vi "Write FTDI.vi"(8 "error in (no error)":errorcluster, 10 "Write STR":string="\u0014", 11 "FTDI Handle In":u32) -> (0 "error out":errorcluster, 2 "FT_Status":u32(ring) items=["FT_OK", "FT_INVALID_HANDLE", "FT_DEVICE_NOT_FOUND", "FT_DEVICE_NOT_OPENED", "FT_IO_ERROR", "FT_INSUFFICIENT_RESOURCES", "FT_INVALID_PARAMETER", "FT_INVALID_BAUD_RATE", "FT_DEVICE_NOT_OPENED_FOR_ERASE", "FT_DEVICE_NOT_OPENED_FOR_WRITE", "FT_FAILED_TO_WRITE_DEVICE", "FT_EEPROM_READ_FAILED", "FT_EEPROM_WRITE_FAILED", "FT_EEPROM_ERASE_FAILED", "FT_EEPROM_NOT_PRESENT", "FT_EEPROM_NOT_PROGRAMMED", "FT_INVALID_ARGS", "FT_NOT_SUPPORTED", "FT_OTHER_ERROR"], 3 "FTDI Handle Out":u32)   [LabVIEW 2011, in "NMR.lvclass"]
uses:
  NMR.lvclass
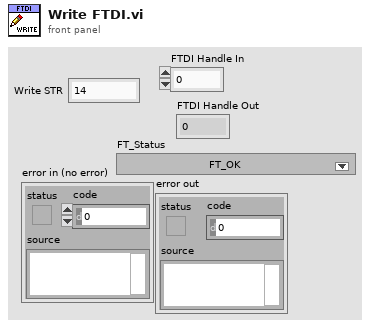
[diagram p1: front panel]
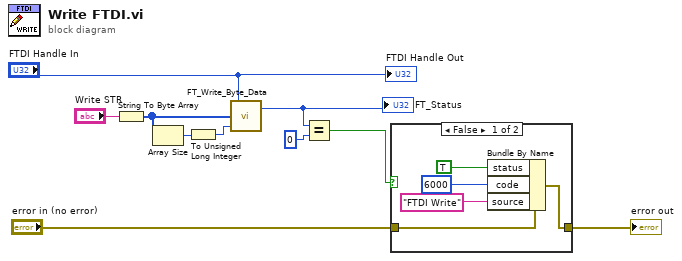
[diagram p0: block diagram]
diagram:
  n1 = String To Byte Array(string="Write STR") -> (unsigned byte array=w7:u8[])
  n2 = Array Size(array=w7) -> (size(s)=w10:i32)
  n3 = To Unsigned Long Integer(number=w10) -> (unsigned 32bit integer=w9:u32)
  n4 = call <instrlib>:"FT_Write_Byte_Data.vi"("Bytes To Write"=w9, "Buffer"=w7, "Handle"="FTDI Handle In") -> ("FT_Status"=w5:u32)  [unwired: 1 out]
  "FT_Status" <- w5
  n5 = Equal?(x=w5, y=u32 0) -> (x = y?=w3:bool)
  n6 = case shown="False" w3 {
    tunnel: [w12 w16] -> w1
    tunnel: "error in (no error)" -> [w15 w16]
    frame False {
      n7 = Bundle By Name(cluster=w15, "status"=TRUE, "code"=6000, "source"="FTDI Write") -> (w12:errorcluster)
    }
    frame True {
    }
  }
  "error out" <- w1
  "FTDI Handle Out" <- "FTDI Handle In"
